vi "setup.vi"(8 "error in (no error)":errorcluster, 11 "Analog_Output in":refnum<class "Analog_Output.lvclass">) -> (0 "error out":errorcluster, 3 "Analog_Output out":refnum<class "Analog_Output.lvclass">)   [LabVIEW 2013, in "Analog_Output.lvclass"]
uses:
  Analog_Output.lvclass
  Analog_Output.lvclass/Analog_Output.ctl
  Experiment/Globals.vi
  <vilib>/DAQmx/create/channels.llb/DAQmx Create Channel (AO-Voltage-Basic).vi
  <vilib>/DAQmx/configure/trigger.llb/DAQmx Start Trigger (Digital Edge).vi
  <vilib>/DAQmx/configure/events/hardwareSignals.llb/DAQmx Export Signal (Most Signals).vi
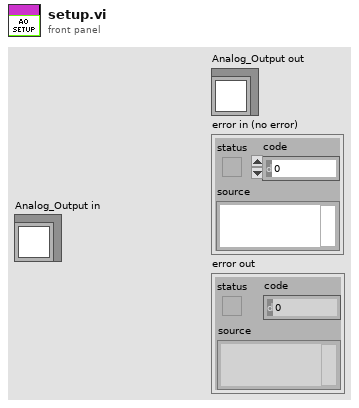
[diagram p1: front panel]
types:
  T1 = typedef "Analog_Output.lvclass/AO_settings.ctl" = cluster{"Enable Analog Out?":bool, "Physical Channel":tag, "Minimum Value":dbl, "Maximum Value":dbl, "Samples per second":dbl, "Total AO Time (seconds)":dbl, "Start Trigger":cluster{"Wait for start trigger?":bool, "source":tag, "edge":i32}, "Analog Output Waveforms (channel, time)":dbl[][], "Export trigger":cluster{"Export Start Trigger?":bool, "output terminal":tag}}
  T2 = cluster{"Wait for start trigger?":bool, "source":tag, "edge":i32}
  T3 = cluster{"Export Start Trigger?":bool, "output terminal":tag}
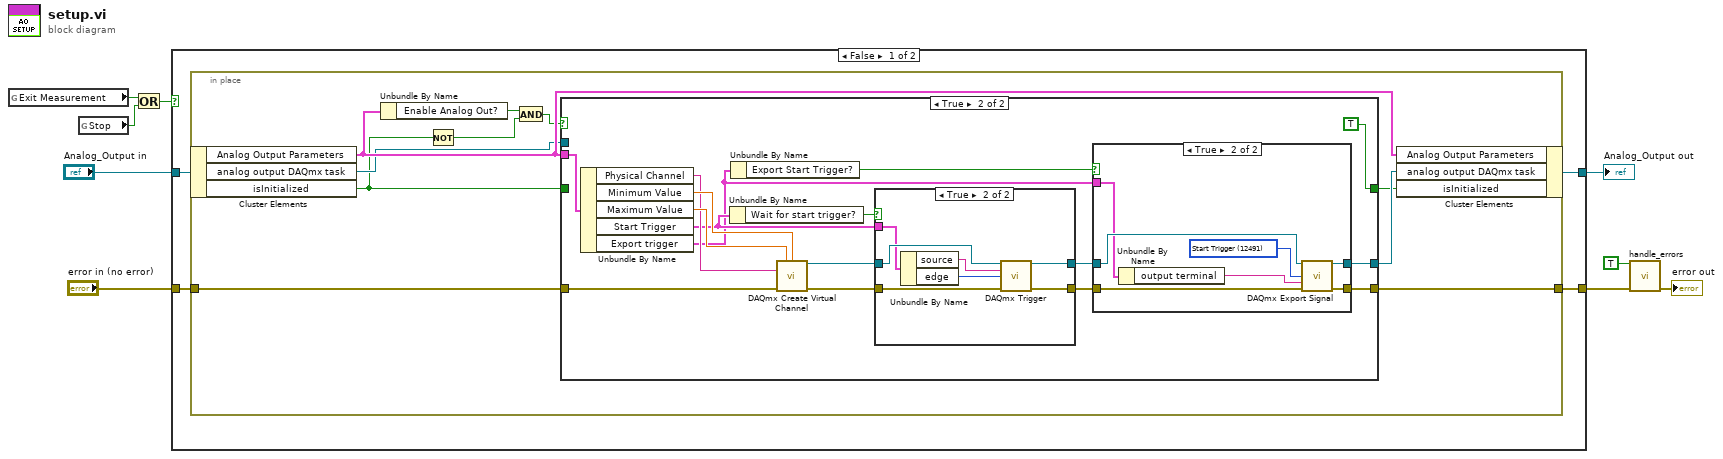
[diagram p0: block diagram]
diagram:
  n1 = global read "Globals.vi" "Exit Measurement"() -> (w8:bool)
  n2 = global read "Globals.vi" "Stop"() -> (w7:bool)
  n3 = Or(x=w8, y=w7) -> (x .or. y?=w5:bool)
  n4 = case shown="False" w5 {
    tunnel: [w12 w62] -> w9
    tunnel: "Analog_Output in" -> [w13 w62]
    tunnel: "error in (no error)" -> [w11 w61]
    tunnel: [w10 w61] -> w2
    frame False {
      n5 = in-place {
        in-place-border: w11 -> [w22]
        in-place-border: [w17] -> w10
        n6 = in-place-cluster #1(w13) -> ("Analog Output Parameters"=w23:T1, "analog output DAQmx task"=w21:refnum<k21>, "isInitialized"=w14:bool)
        n7 = Unbundle By Name(w23) -> ("Enable Analog Out?"=w19:bool)
        n8 = Not(x=w14) -> (.not. x?=w20:bool)
        n9 = And(x=w19, y=w20) -> (x .and. y?=w16:bool)
        n10 = case shown="True" w16 {
          tunnel: w22 -> [w26 w42]
          tunnel: [w26 w32] -> w17
          tunnel: [w25 w31] -> w18
          tunnel: w23 -> [_ w41]
          tunnel: w21 -> [w25 _]
          tunnel: [w24 TRUE ("isInitialized")] -> w15
          tunnel: w14 -> [w24 _]
          frame False {
          }
          frame True {
            n11 = Unbundle By Name(w41) -> ("Physical Channel"=w38:tag, "Minimum Value"=w40:dbl, "Maximum Value"=w39:dbl, "Start Trigger"=w37:T2, "Export trigger"=w27:T3)
            n12 = Unbundle By Name(w37) -> ("Wait for start trigger?"=w36:bool)
            n13 = Unbundle By Name(w27) -> ("Export Start Trigger?"=w28:bool)
            n14 = call-poly <vilib>:"DAQmx Create Virtual Channel.vi"("maximum value"=w39, "minimum value"=w40, "physical channels"=w38, "error in"=w42) -> ("task out"=w34:refnum<k21>, "error out"=w35:errorcluster)  [unwired: 10 in]
            n15 = case shown="True" w36 {
              tunnel: [w53 w60] -> w33
              tunnel: [w52 w59] -> w30
              tunnel: w34 -> [w52 w58]
              tunnel: w35 -> [w53 w57]
              tunnel: w37 -> [_ w56]
              frame False {
              }
              frame True {
                n16 = Unbundle By Name(w56) -> ("source"=w55:tag, "edge"=w54:i32)
                n17 = call-poly <vilib>:"DAQmx Trigger.vi"("task/channels in"=w58, "source"=w55, "edge"=w54, "error in"=w57) -> ("task out"=w59:refnum<k21>, "error out"=w60:errorcluster)  [unwired: 10 in]
              }
            }
            n18 = case shown="True" w28 {
              tunnel: w33 -> [w43 w50]
              tunnel: [w43 w49] -> w32
              tunnel: [w44 w48] -> w31
              tunnel: w30 -> [w44 w47]
              tunnel: w27 -> [_ w46]
              frame False {
              }
              frame True {
                w51 = 12491 items=["AI Convert Clock"=12484, "10MHz Reference Clock"=12536, "20MHz Timebase Clock"=12486, "Sample Clock"=12487, "Advance Trigger"=12488, "Reference Trigger"=12490, "Start Trigger"=12491, "Advance Complete Event"=12492, "AI Hold Complete Event"=12493, "Counter Output Event"=12494, "Change Detection Event"=12511, "Watchdog Timer Expired Event"=12512] ("signal")
                n19 = Unbundle By Name(w46) -> ("output terminal"=w45:tag)
                n20 = call-poly <vilib>:"DAQmx Export Signal.vi"("task/channels in"=w47, "signal"=w51, "output terminal"=w45, "error in"=w50) -> ("task out"=w48:refnum<k21>, "error out"=w49:errorcluster)  [unwired: 10 in]
              }
            }
          }
        }
        n21 = in-place-cluster #1("Analog Output Parameters"=w23, "analog output DAQmx task"=w18, "isInitialized"=w15) -> (w12:refnum<class "Analog_Output.lvclass">)
      }
    }
    frame True {
    }
  }
  "Analog_Output out" <- w9
  n22 = call "handle_errors.vi"("Exit Operation"=TRUE, "error in (no error)"=w2) -> ("error out"=→"error out":errorcluster)  [unwired: 13 in]
